vi "Check Disable Mode.vi"(4 "Vesta in":refnum<queue>, 6 "Timer in":refnum<queue>, 8 "error in (no error)":errorcluster, 11 "Data Cluster in":T1 {"VestaTemperature"."Water Heater Temp (°F)" min=32 max=203}) -> (0 "error out":errorcluster, 3 "Data Cluster Output":T1 {"VestaTemperature"."Water Heater Temp (°F)" min=32 max=203})   [LabVIEW 2023]
uses:
  Message Queue/Message Cluster.ctl
  Message Queue/Message Queue.lvlib
  Drivers/Resideo Gas Valve/Type Definitions/Vesta Info.ctl
  controls/Burner Duty Cycle.ctl
  Drivers/Resideo Gas Valve/Type Definitions/Temperature Control.ctl
  controls/UI Data.ctl
  controls/Timer Application Cluster.ctl
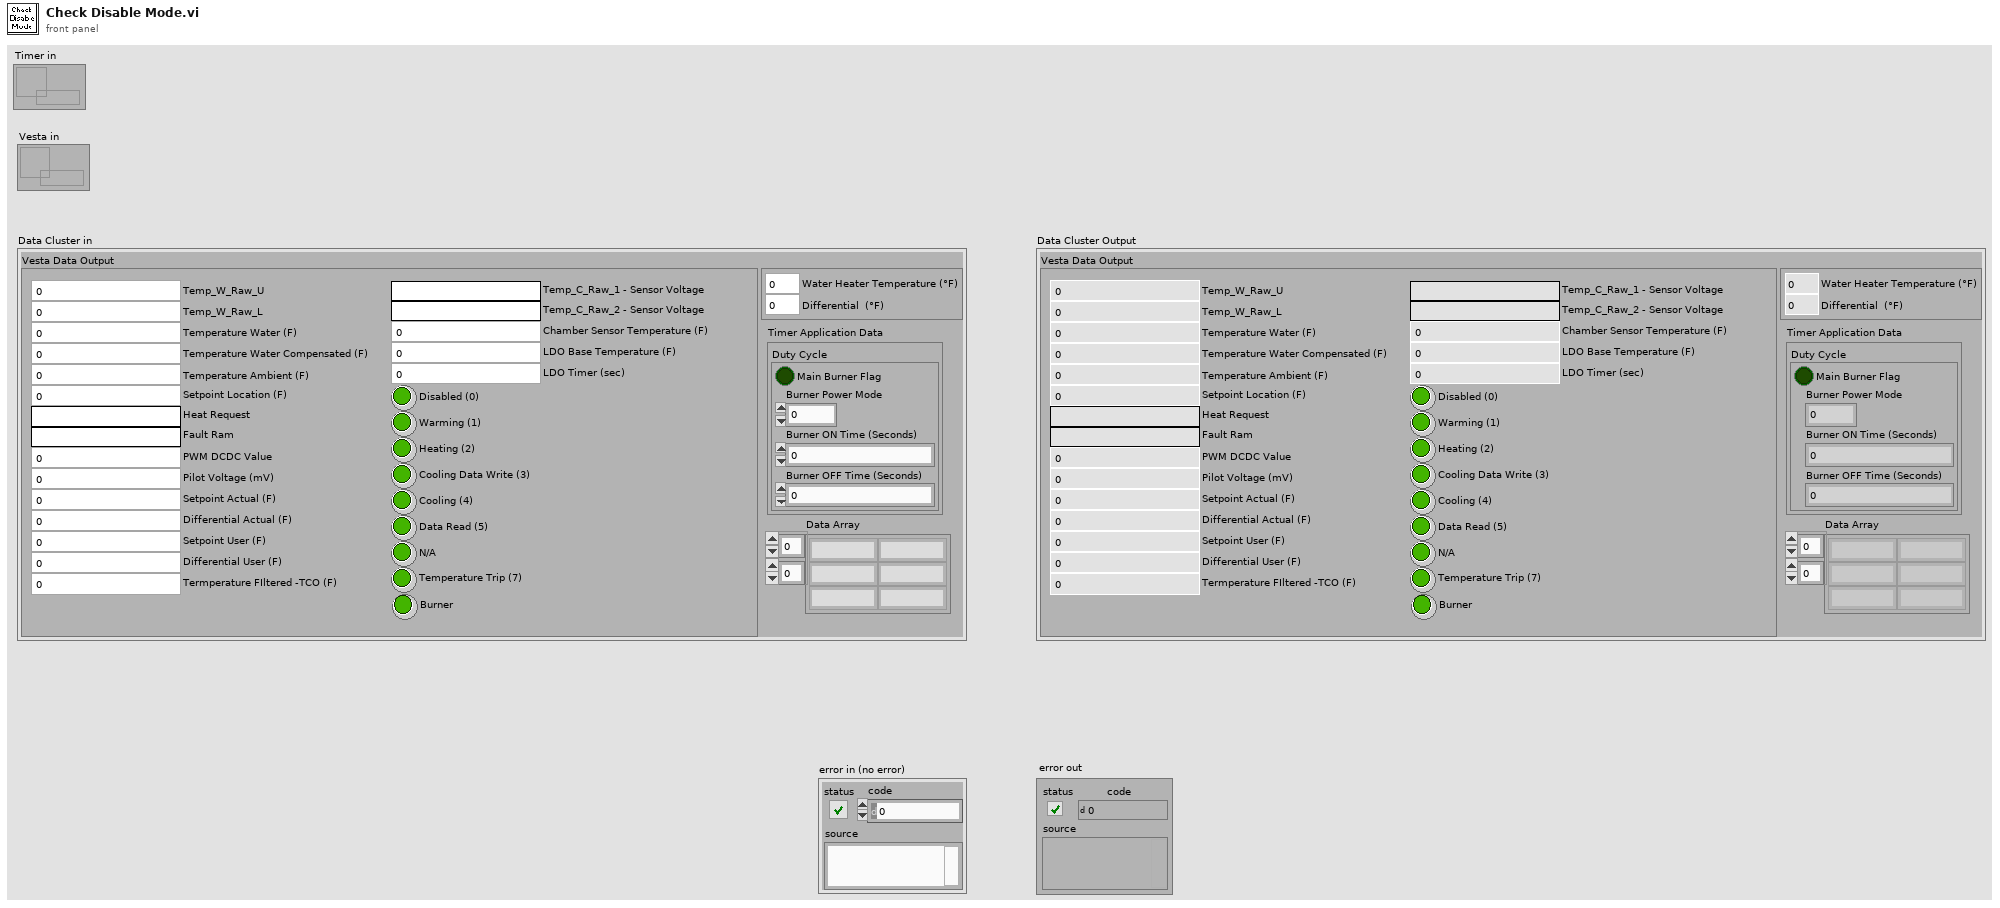
[diagram p1: front panel]
types:
  T1 = typedef "UI Data.ctl" = cluster{"Vesta Data Output":T2, "VestaTemperature":T3, "Timer Application Data":T4, "Data Array":string[][]}
  T2 = typedef "Vesta Info.ctl" = cluster{"Temp_W_Raw_U":u16, "Temp_W_Raw_L":u16, "Temperature Water (F)":dbl, "Temperature Water Compensated (F)":dbl, "Temperature Ambient (F)":dbl, "Setpoint Location (F)":dbl, "Heat Request":string, "Fault Ram":string, "PWM DCDC Value":u16, "Pilot Voltage (mV)":dbl, "Setpoint Actual (F)":dbl, "Differential Actual (F)":dbl, "Setpoint User (F)":dbl, "Differential User (F)":dbl, "Termperature FIltered -TCO (F)":dbl, "Temp_C_Raw_1 - Sensor Voltage":string, "Temp_C_Raw_2 - Sensor Voltage":string, "Chamber Sensor Temperature (F)":dbl, "LDO Base Temperature (F)":dbl, "LDO Timer (sec)":i16, "Disabled (0)":bool, "Warming (1)":bool, "Heating (2)":bool, "Cooling Data Write (3)":bool, "Cooling (4)":bool, "Data Read (5)":bool, "N/A":bool, "Temperature Trip (7)":bool, "Burner":bool}
  T3 = typedef "Temperature Control.ctl" = cluster{"Water Heater Temp (°F)":u16, "Differential  (°F)":dbl}
  T4 = typedef "Timer Application Cluster.ctl" = cluster{"Duty Cycle":T5}
  T5 = typedef "Burner Duty Cycle.ctl" = cluster{"Burner ON Time (Seconds)":dbl, "Burner OFF Time (Seconds)":dbl, "Main Burner Flag":bool, "Burner Power Mode":u8}
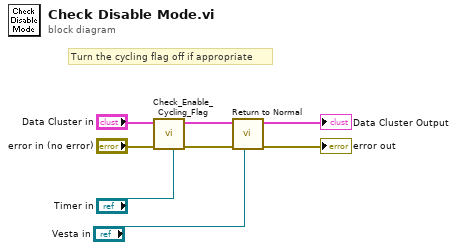
[diagram p0: block diagram]
diagram:
  # "Turn the cycling flag off if appropriate"
  n1 = call "Check_Enable_Cycling_Flag.vi"("Send_Vesta_Message"="Timer in", "error in (no error)"="error in (no error)", "Data Cluster in"="Data Cluster in") -> ("error out"=w7:errorcluster, "Data Cluster out"=w1:T1)  [unwired: 6 in, 1 out]
  n2 = call "Return to Normal.vi"(6:"Vesta in", "error in (no error)"=w7, "Data Cluster in"=w1) -> ("error out"=→"error out":errorcluster, "Data Cluster Output"=→"Data Cluster Output":T1)  [unwired: 6 in, 1 out]
